vi "Floor_Panel_Heater_Control.vi"(1 "Ch Names":string[](array[string]), 2 "Values":dbl[](array[numeric]) format="%.2f") -> ()   [LabVIEW 2010]
uses:
  ADAM_Global.vi
  <vilib>/Analysis/NI_AALPro.lvlib
  <vilib>/Analysis/NI_AALBase.lvlib
panel:
  in  "Total History (s)":i32=80
  out "Proportional Term":dbl format="%#.1f"
  out "Control Sum":dbl format="%#.1f"
  out "Differential Term":dbl format="%#.1f"
  in  "Derivative History (s)":i32=15
  out "Integral Term":dbl format="%#.1f"
  in  "Kp":dbl=6.0 format="%.2f"
  in  "Kd":dbl=150.0 format="%.2f"
  in  "Ki":dbl=0.05 format="%.2f"
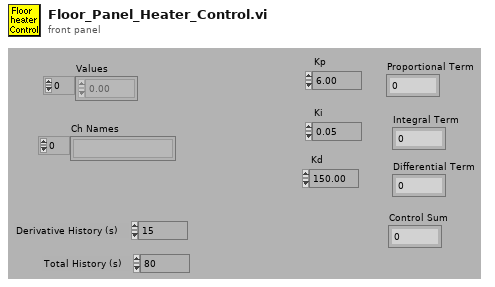
[diagram p1: front panel]
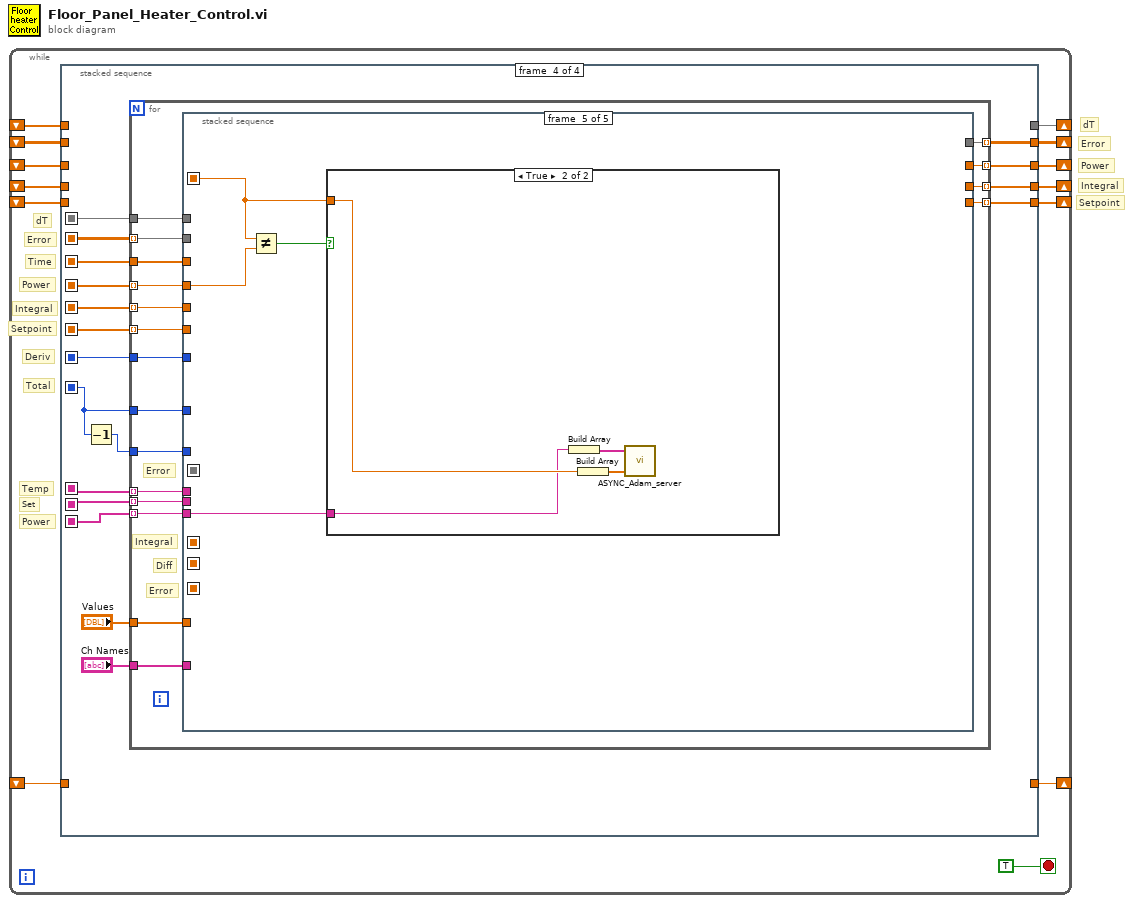
[diagram p0: block diagram]
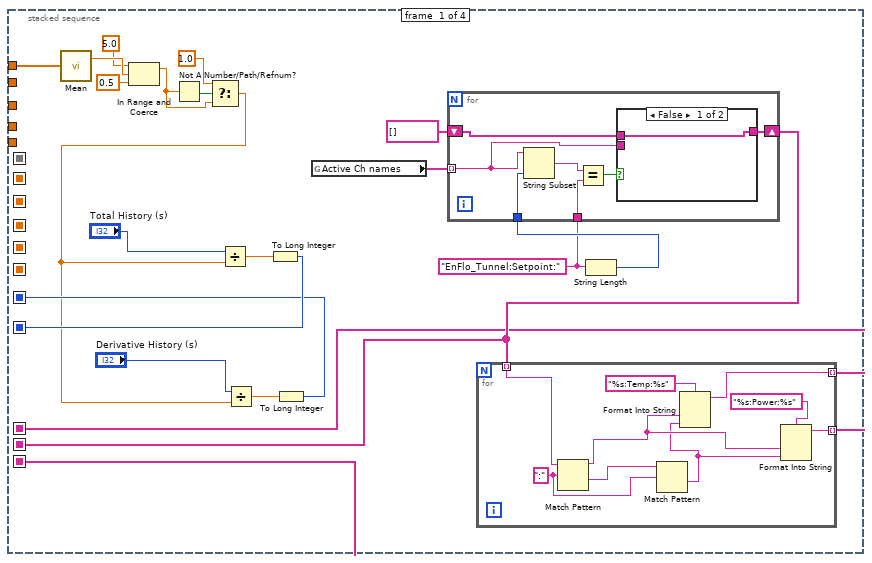
[diagram p2: hidden frame]
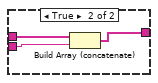
[diagram p3: hidden frame]
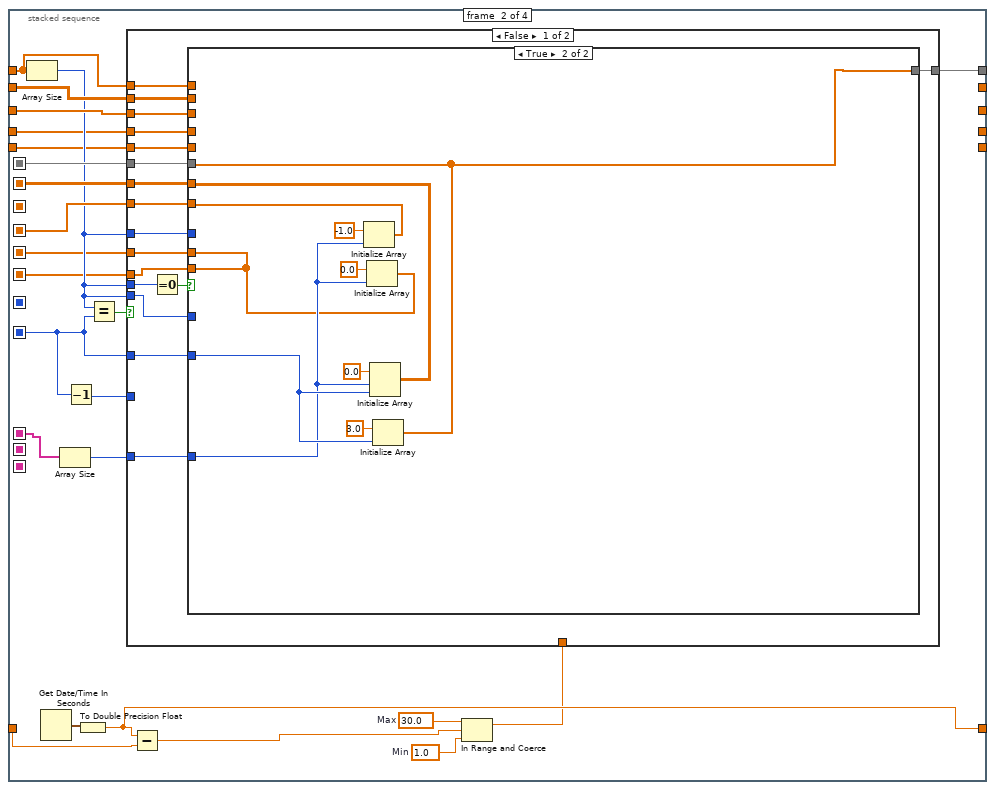
[diagram p4: hidden frame]
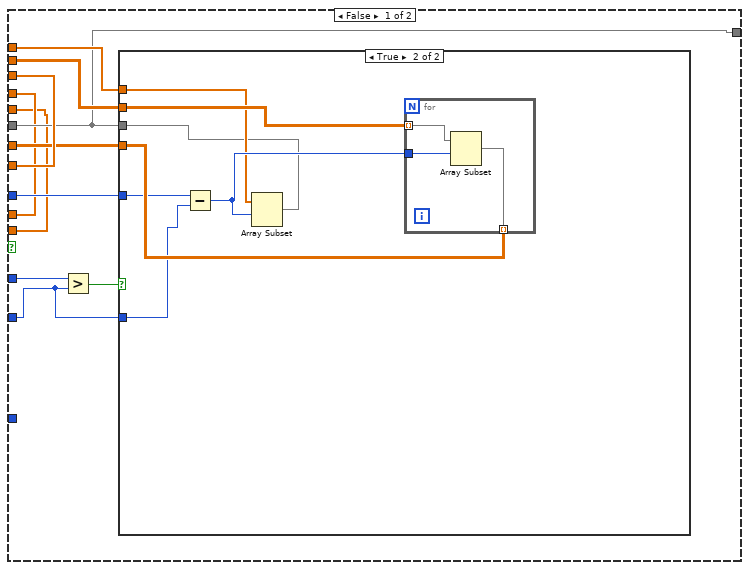
[diagram p5: hidden frame]
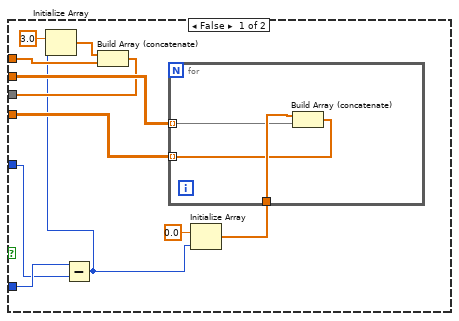
[diagram p6: hidden frame]
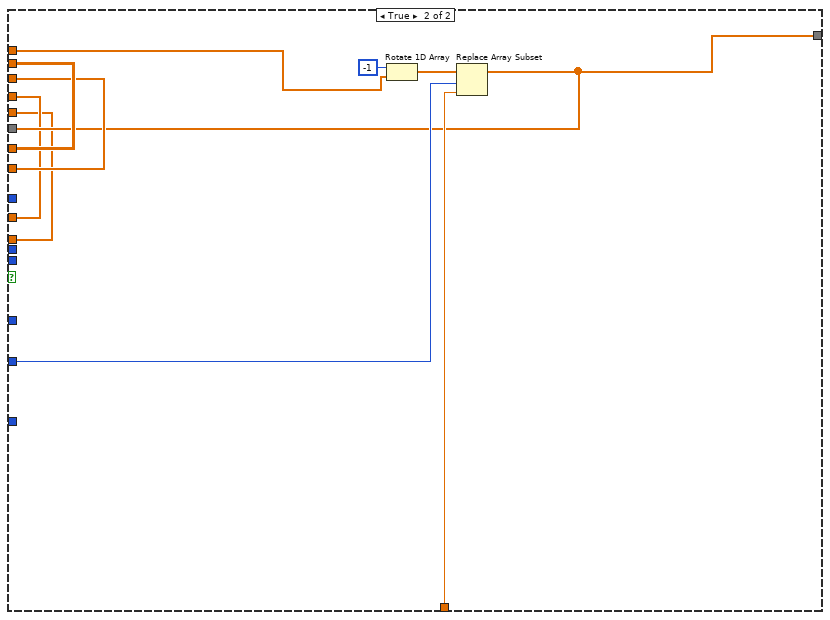
[diagram p7: hidden frame]
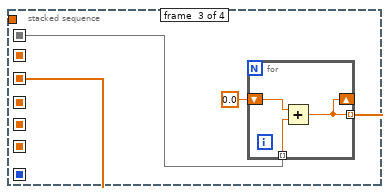
[diagram p8: hidden frame]
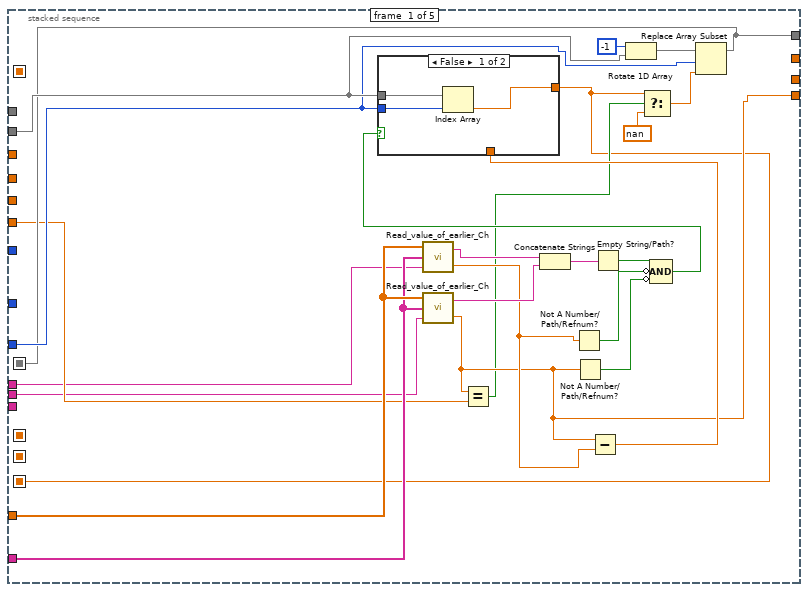
[diagram p9: hidden frame]
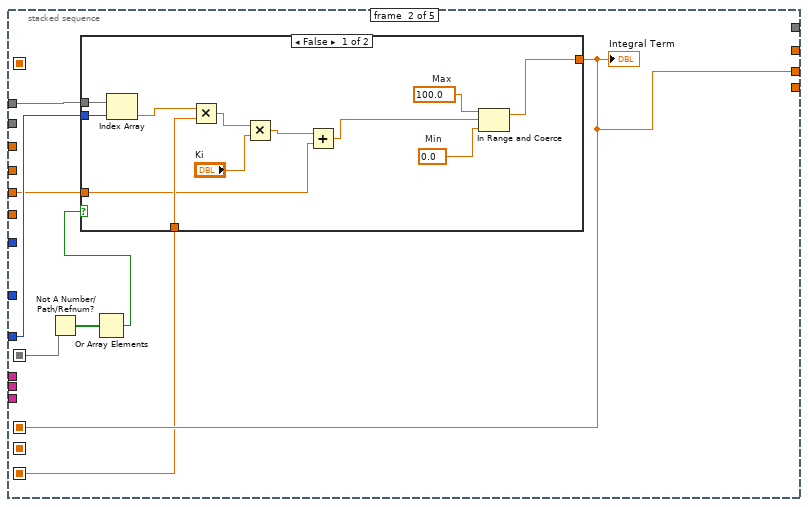
[diagram p11: hidden frame]
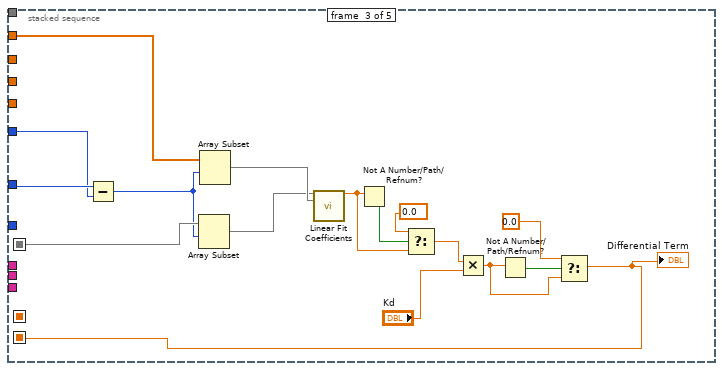
[diagram p13: hidden frame]
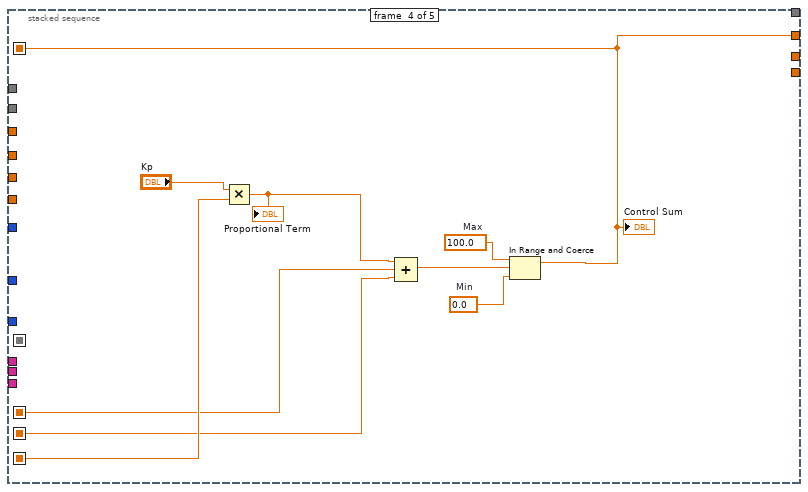
[diagram p14: hidden frame]
diagram:
  # "Setpoint"
  # "Power"
  # "Integral"
  # "Error"
  # "dT"
  n1 = while {
    shift-right: [w11] -> _
    shift-left: _ -> [w12]
    shift-right: [w7] -> _
    shift-left: _ -> [w10]
    shift-right: [w9] -> _
    shift-left: _ -> [w8]
    shift-right: [w5] -> _
    shift-left: _ -> [w6]
    shift-right: [w3] -> _
    shift-left: _ -> [w4]
    shift-right: [w1] -> _
    shift-left: _ -> [w2]
    stop <- TRUE stop-if-true
    # "Power"
    # "Set"
    # "Temp"
    # "Total"
    # "Deriv"
    # "Setpoint"
    # "Integral"
    # "Power"
    # "Time"
    # "Error"
    # "dT"
    n2 = stacked-sequence {
      seq-local: [_ w77 _ _] -> [_ _ w152 w170]
      seq-local: [_ w67 _ _] -> [_ _ _ w172]
      seq-local: [_ _ w151 _] -> [_ _ _ w169]
      seq-local: [_ w65 _ _] -> [_ _ _ w167]
      seq-local: [_ w63 _ _] -> [_ _ _ w165]
      seq-local: [_ w61 _ _] -> [_ _ _ w163]
      seq-local: [w31 _ _ _] -> [_ w56 _ w162]
      seq-local: [w28 _ _ _] -> [_ _ _ w160]
      seq-local: [w14 _ _ _] -> [_ w55 _ w159]
      seq-local: [w16 _ _ _] -> [_ _ _ w158]
      seq-local: [w15 _ _ _] -> [_ _ _ w157]
      tunnel: w12 -> [w34 w59 _ _]
      tunnel: [_ w72 _ _] -> w11
      tunnel: w10 -> [_ w76 _ _]
      tunnel: [_ w73 _ _] -> w9
      tunnel: w8 -> [_ w74 _ _]
      tunnel: [_ _ _ w171] -> w7
      tunnel: w6 -> [_ w66 _ _]
      tunnel: [_ _ _ w168] -> w5
      tunnel: w4 -> [_ w62 _ _]
      tunnel: [_ _ _ w166] -> w3
      tunnel: w2 -> [_ w60 _ _]
      tunnel: [_ _ _ w164] -> w1
      frame #0 {
        w18 = "EnFlo_Tunnel:Setpoint:"
        n3 = call <vilib>:"Mean.vi"("X"=w34) -> ("mean"=w27:dbl)  [unwired: 1 out]
        n4 = In Range and Coerce(upper limit=5.0, x=w27, lower limit=0.5) -> (coerced(x)=w23:dbl)  [unwired: 1 out]
        n5 = Not A Number/Path/Refnum?(number/path/refnum=w23) -> (NaN/Path/Refnum?=w24:bool)
        n6 = Select(t=1.0, s=w24, f=w23) -> (s? t:f=w21:dbl)
        n7 = Divide(x="Total History (s)", y=w21) -> (x/y=w32:dbl)
        n8 = Divide(x="Derivative History (s)", y=w21) -> (x/y=w30:dbl)
        n9 = To Long Integer(number=w32) -> (32bit integer=w31:i32)
        n10 = To Long Integer(number=w30) -> (32bit integer=w28:i32)
        n11 = global read "ADAM_Global.vi" "Active Ch names"() -> (w20:string[])
        n12 = String Length(string=w18) -> (length=w19:i32)
        n13 = for {
          shift-right: [w35] -> w16
          shift-left: string[] [] -> [w37]
          tunnel: w20 -> [w36] mode=indexing
          tunnel: w19 -> [w41]
          tunnel: w18 -> [w40]
          n14 = String Subset(string=w36, length (rest)=w41) -> (substring=w39:string)  [unwired: 1 out]
          n15 = Equal?(x=w39, y=w40) -> (x = y?=w38:bool)
          n16 = case shown="False" w38 {
            tunnel: w37 -> [w42 w45]
            tunnel: w36 -> [_ w44]
            tunnel: [w42 w43] -> w35
            frame False {
            }
            frame True {
              n17 = Build Array (concatenate)(w45, w44) -> (w43:string[])
            }
          }
        }
        n18 = for {
          tunnel: w16 -> [w46] mode=indexing
          tunnel: [w47] -> w15 mode=indexing
          tunnel: [w48] -> w14 mode=indexing
          w53 = ":" ("regular expression")
          n19 = Match Pattern(string=w46, regular expression=w53) -> (before substring=w50:string, after substring=w54:string)  [unwired: 3 out]
          n20 = Match Pattern(string=w54, regular expression=w53) -> (after substring=w49:string)  [unwired: 4 out]
          n21 = Format Into String(format string="%s:Temp:%s", w50, w49) -> (resulting string=w48:string)  [unwired: 2 in, 1 out]
          n22 = Format Into String(format string="%s:Power:%s", w50, w49) -> (resulting string=w47:string)  [unwired: 2 in, 1 out]
        }
      }
      frame #1 {
        w71 = 1.0  # Min
        w70 = 30.0  # Max
        n23 = Array Size(array=w59) -> (size(s)=w64:i32)
        n24 = Get Date/Time In Seconds() -> (seconds since 1Jan1904=w75:timestamp)
        n25 = Array Size(array=w55) -> (size(s)=w58:i32)
        n26 = Decrement(x=w56) -> (x-1=w57:i32)
        n27 = To Double Precision Float(number=w75) -> (double precision float=w73:dbl)
        n28 = Equal?(x=w64, y=w56) -> (x = y?=w78:bool)
        n29 = Subtract(x=w73, y=w74) -> (x-y=w69:dbl)
        n30 = In Range and Coerce(upper limit=w70, x=w69, lower limit=w71) -> (coerced(x)=w68:dbl)  [unwired: 1 out]
        n31 = case shown="False" w78 {
          tunnel: [w91 w143] -> w77
          tunnel: w59 -> [w84 w148]
          tunnel: [w89 w150] -> w67
          tunnel: w76 -> [w92 w150]
          tunnel: w64 -> [w95 _]
          tunnel: w56 -> [w93 _]
          tunnel: w68 -> [_ w146]
          tunnel: [w83 w143] -> w72
          tunnel: w57 -> [_ w145]
          tunnel: w58 -> [w90 _]
          tunnel: w66 -> [w87 w144]
          tunnel: [w88 w144] -> w65
          tunnel: w64 -> [w86 _]
          tunnel: w64 -> [w85 _]
          tunnel: [w82 w142] -> w63
          tunnel: w62 -> [w81 w142]
          tunnel: [w80 w141] -> w61
          tunnel: w60 -> [w79 w141]
          frame False {
            n32 = Equal To 0?(x=w95) -> (x = 0?=w94:bool)
            n33 = case shown="True" w94 {
              tunnel: w93 -> [w103 w138]
              tunnel: w92 -> [w102 _]
              tunnel: [w98 w134] -> w91
              tunnel: w90 -> [_ w132]
              tunnel: [w101 w137] -> w89
              tunnel: [w106 w135] -> w88
              tunnel: w87 -> [w106 _]
              tunnel: w86 -> [w105 _]
              tunnel: w85 -> [w100 _]
              tunnel: w84 -> [w99 _]
              tunnel: [w98 w134] -> w83
              tunnel: [w97 w131] -> w82
              tunnel: w81 -> [w97 _]
              tunnel: [w96 w131] -> w80
              tunnel: w79 -> [w96 _]
              frame False {
                n34 = Greater?(x=w105, y=w103) -> (0:w104:bool)
                n35 = case shown="True" w104 {
                  tunnel: w103 -> [w117 w125]
                  tunnel: w102 -> [w113 w127]
                  tunnel: [w112 w126] -> w101
                  tunnel: w100 -> [w116 w124]
                  tunnel: w99 -> [w109 w122]
                  tunnel: [w108 w121] -> w98
                  frame False {
                    n36 = Subtract(x=w117, y=w116) -> (x-y=w107:i32)
                    n37 = Initialize Array(3.0 ("element"), w107) -> (w110:dbl[])
                    n38 = Build Array (concatenate)(w110, w109) -> (w108:dbl[])
                    n39 = Initialize Array(0.0 ("element"), w107) -> (w114:dbl[])
                    n40 = for {
                      tunnel: w114 -> [w120]
                      tunnel: w113 -> [w119] mode=indexing
                      tunnel: [w118] -> w112 mode=indexing
                      n41 = Build Array (concatenate)(w120, w119) -> (w118:dbl[])
                    }
                  }
                  frame True {
                    n42 = Subtract(x=w124, y=w125) -> (x-y=w123:i32)
                    n43 = Array Subset(array=w122, index=w123) -> (w121:dbl[])  [unwired: 1 in]
                    n44 = for {
                      tunnel: w127 -> [w130] mode=indexing
                      tunnel: [w129] -> w126 mode=indexing
                      tunnel: w123 -> [w128]
                      n45 = Array Subset(array=w130, index=w128) -> (w129:dbl[])  [unwired: 1 in]
                    }
                  }
                }
              }
              frame True {
                n46 = Initialize Array(-1.0 ("element"), w132) -> (w135:dbl[])
                n47 = Initialize Array(0.0 ("element"), w132) -> (w131:dbl[])
                n48 = Initialize Array(0.0 ("element"), w132, w138) -> (w137:dbl[][])
                n49 = Initialize Array(3.0 ("element"), w138) -> (w134:dbl[])
              }
            }
          }
          frame True {
            n50 = Rotate 1D Array(1:w148, 2:-1 ("n")) -> (0:w147:dbl[])
            n51 = Replace Array Subset(array=w147, new element=w146, index=w145) -> (w143:dbl[])
          }
        }
      }
      frame #2 {
        n52 = for {
          shift-right: [w154] -> _
          shift-left: 0.0 ("element") -> [w156]
          tunnel: w152 -> [w155] mode=indexing
          tunnel: [w154] -> w151 mode=indexing
          n53 = Add(x=w156, y=w155) -> (x+y=w154:dbl)
        }
      }
      frame #3 {
        n54 = Decrement(x=w162) -> (x-1=w161:i32)
        n55 = for {
          tunnel: "Values" -> [w192]
          tunnel: "Ch Names" -> [w191]
          tunnel: [w190] -> w171 mode=indexing
          tunnel: w172 -> [w189] mode=indexing
          tunnel: w161 -> [w188]
          tunnel: w170 -> [w187]
          tunnel: w162 -> [w186]
          tunnel: w169 -> [w185]
          tunnel: [w184] -> w168 mode=indexing
          tunnel: w167 -> [w183] mode=indexing
          tunnel: [w182] -> w166 mode=indexing
          tunnel: w165 -> [w181] mode=indexing
          tunnel: [w180] -> w164 mode=indexing
          tunnel: w163 -> [w179] mode=indexing
          tunnel: w160 -> [w178]
          tunnel: w159 -> [w177] mode=indexing
          tunnel: w158 -> [w176] mode=indexing
          tunnel: w157 -> [w175] mode=indexing
          # "Integral"
          # "Error"
          # "Error"
          # "Diff"
          n56 = stacked-sequence {
            seq-local: [_ _ w251 _ _] -> [_ _ _ w262 _]
            seq-local: [w196 _ _ _ _] -> [_ w225 _ w266 _]
            seq-local: [w201 _ _ _ _] -> [_ w223 w245 _ _]
            seq-local: [_ w228 _ _ _] -> [_ _ _ w263 _]
            seq-local: [_ _ _ w258 _] -> [_ _ _ _ w268]
            tunnel: w192 -> [w216 _ _ _ _]
            tunnel: w191 -> [w215 _ _ _ _]
            tunnel: [w201 _ _ _ _] -> w190
            tunnel: w189 -> [w203 _ _ _ _]
            tunnel: w188 -> [w202 w227 _ _ _]
            tunnel: w187 -> [_ w226 _ _ _]
            tunnel: w186 -> [_ _ w248 _ _]
            tunnel: w185 -> [_ _ w247 _ _]
            tunnel: [_ _ _ w258 _] -> w184
            tunnel: w183 -> [_ _ _ _ w270]
            tunnel: [_ w228 _ _ _] -> w182
            tunnel: w181 -> [_ w224 _ _ _]
            tunnel: [w200 _ _ _ _] -> w180
            tunnel: w179 -> [w199 _ _ _ _]
            tunnel: w178 -> [_ _ w242 _ _]
            tunnel: w177 -> [w194 _ _ _ _]
            tunnel: w176 -> [w193 _ _ _ _]
            tunnel: w175 -> [_ _ _ _ w267]
            frame #0 {
              n57 = call "Read_value_of_earlier_Ch.vi"("Desired Ch to Read"=w194, "Ch names"=w215, "Present scan array"=w216) -> ("Value"=w208:dbl, "Scan comment"=w214:string)  [unwired: 1 in]
              n58 = call "Read_value_of_earlier_Ch.vi"("Desired Ch to Read"=w193, "Ch names"=w215, "Present scan array"=w216) -> ("Value"=w200:dbl, "Scan comment"=w213:string)  [unwired: 1 in]
              n59 = Equal?(x=w200, y=w199) -> (x = y?=w198:bool)
              n60 = Concatenate Strings(w214, w213) -> (w212:string)
              n61 = Not A Number/Path/Refnum?(number/path/refnum=w208) -> (NaN/Path/Refnum?=w210:bool)
              n62 = Not A Number/Path/Refnum?(number/path/refnum=w200) -> (NaN/Path/Refnum?=w209:bool)
              n63 = Subtract(x=w200, y=w208) -> (x-y=w206:dbl)
              n64 = Empty String/Path?(string/path=w212) -> (empty?=w211:bool)
              n65 = Rotate 1D Array(1:w203, 2:-1 ("n")) -> (0:w204:dbl[])
              n66 = Compound Arithmetic op=AND(w211, invert w210, invert w209) -> (w207:bool)
              n67 = case shown="False" w207 {
                tunnel: w202 -> [w219 _]
                tunnel: w203 -> [w218 _]
                tunnel: [w217 w220] -> w196
                tunnel: w206 -> [_ w220]
                frame False {
                  n68 = Index Array(array=w218, index=w219) -> (element=w217:dbl)
                }
                frame True {
                }
              }
              n69 = Select(t=w196, s=w198, f=nan) -> (s? t:f=w197:dbl)
              n70 = Replace Array Subset(array=w204, new element=w197, index=w202) -> (w201:dbl[])
            }
            frame #1 {
              n71 = Not A Number/Path/Refnum?(number/path/refnum=w223) -> (NaN/Path/Refnum?=w222:bool[])
              n72 = Or Array Elements(Boolean array=w222) -> (logical OR=w221:bool)
              n73 = case shown="False" w221 {
                tunnel: [w237 w241] -> w228
                tunnel: w227 -> [w236 _]
                tunnel: w226 -> [w235 _]
                tunnel: w225 -> [w233 _]
                tunnel: w224 -> [w231 w241]
                frame False {
                  w240 = 0.0  # Min
                  w238 = 100.0  # Max
                  n74 = Index Array(array=w235, index=w236) -> (element=w234:dbl)
                  n75 = Multiply(x=w234, y=w233) -> (x*y=w232:dbl)
                  n76 = Multiply(x=w232, y="Ki") -> (x*y=w230:dbl)
                  n77 = Add(x=w230, y=w231) -> (x+y=w229:dbl)
                  n78 = In Range and Coerce(upper limit=w238, x=w229, lower limit=w240) -> (coerced(x)=w237:dbl)  [unwired: 1 out]
                }
                frame True {
                }
              }
              "Integral Term" <- w228
            }
            frame #2 {
              n79 = Subtract(x=w248, y=w242) -> (x-y=w243:i32)
              n80 = Array Subset(array=w245, index=w243) -> (w244:dbl[])  [unwired: 1 in]
              n81 = Array Subset(array=w247, index=w243) -> (w246:dbl[])  [unwired: 1 in]
              n82 = call <vilib>:"Linear Fit Coefficients.vi"("Y"=w244, "X"=w246) -> ("slope"=w257:dbl)  [unwired: 3 in, 10 out]
              n83 = Not A Number/Path/Refnum?(number/path/refnum=w257) -> (NaN/Path/Refnum?=w255:bool)
              n84 = Select(t=0.0 ("f"), s=w255, f=w257) -> (s? t:f=w254:dbl)
              n85 = Multiply(x=w254, y="Kd") -> (x*y=w250:dbl)
              n86 = Not A Number/Path/Refnum?(number/path/refnum=w250) -> (NaN/Path/Refnum?=w252:bool)
              n87 = Select(t=0.0, s=w252, f=w250) -> (s? t:f=w251:dbl)
              "Differential Term" <- w251
            }
            frame #3 {
              w261 = 0.0  # Min
              w260 = 100.0  # Max
              n88 = Multiply(x="Kp", y=w266) -> (x*y=w264:dbl)
              "Proportional Term" <- w264
              n89 = Compound Arithmetic op=ADD(w264, w263, w262) -> (w259:dbl)
              n90 = In Range and Coerce(upper limit=w260, x=w259, lower limit=w261) -> (coerced(x)=w258:dbl)  [unwired: 1 out]
              "Control Sum" <- w258
            }
            frame #4 {
              n91 = Not Equal?(x=w268, y=w270) -> (x != y?=w269:bool)
              n92 = case shown="True" w269 {
                tunnel: w268 -> [_ w272]
                tunnel: w267 -> [_ w271]
                frame False {
                }
                frame True {
                  n93 = Build Array(w271) -> (w273:string[])
                  n94 = Build Array(w272) -> (w274:dbl[])
                  n95 = call "ASYNC_Adam_server.vi"("Values"=w274, "Channel Names"=w273) -> ()  [unwired: 1 in, 3 out]
                }
              }
            }
          }
        }
      }
    }
  }
